vi "RST.vi"(0 "System no.":i32=1 min=1 max=4 step=1, 2 "Axes to be restored":string[](array[string]), 3 "All axes?":bool, 4 "Axis identifier?":bool=TRUE, 5 "error in":errorcluster) -> (19 "error out":errorcluster)   [LabVIEW 2020]
doc: "Restores parameters or resets E-816 master unit.\n\nC-702: If All axes = TRUE, then Axis identifier must be TRUE. Restores last saved stage configuration in volatile memeory (RAM) for any of the specified axes. Loads back the stage configuration (can be modified with CST) and the motion parameters (can be modified with SPA) which were last saved with SAV. \n\nC-848: If All axes = TRUE, then Axis identifier must be TRUE. Restores parameters of any of the specified axes which have been modified using SPA command to values from last SAV.\nC-880: If All axes = TRUE, then Axis identifier must be TRUE. Restores parameters of any of the specified axes which have been modified using SPA command to values from last SAV. \nE-816: All axes = TRUE, Axis identifier = FALSE; this command affects the master unit only. (Resets the master unit.)"
panel:
  # "Restores parameters or resets E-816 master unit."
  # "If all axes: use"
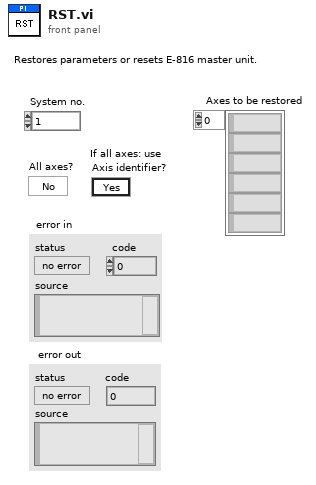
[diagram p1: front panel]
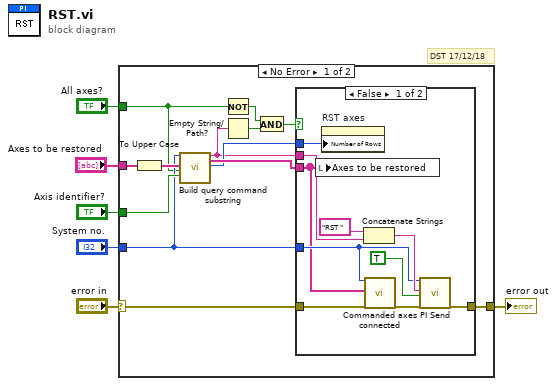
[diagram p0: block diagram]
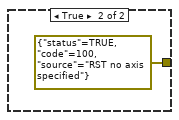
[diagram p2: hidden frame]
diagram:
  # "DST 17/12/18"
  n1 = case shown="No Error" "error in" {
    selector: "error in" -> [w10 w31]
    tunnel: "Axes to be restored" -> [w19 _]
    tunnel: "Axis identifier?" -> [w17 _]
    tunnel: "System no." -> [w16 _]
    tunnel: "All axes?" -> [w13 _]
    tunnel: [w11 w31] -> w2
    frame No Error {
      n2 = To Upper Case(1:w19) -> (0:w18:string[])
      n3 = call "Build query command substring.vi"("System no."=w16, "Axes to query in"=w18, "Query\nAll axes?"=w13, "For all axes: use\nAxis identifier?"=w17) -> ("Command substring"=w7:string, "Axes to query out"=w15:string[], "Number of rows"=w14:u32)  [unwired: 2 in, 11 out]
      n4 = Not(x=w13) -> (.not. x?=w12:bool)
      n5 = Empty String/Path?(string/path=w7) -> (empty?=w8:bool)
      n6 = And(x=w12, y=w8) -> (x .and. y?=w9:bool)
      n7 = case shown="False" w9 {
        tunnel: w7 -> [w26 _]
        tunnel: w16 -> [w25 _]
        tunnel: w15 -> [w24 _]
        tunnel: w14 -> [w22 _]
        tunnel: [w21 errorcluster {"status"=TRUE, "code"=100, "source"="RST no axis specified"} ("error out")] -> w11
        tunnel: w10 -> [w20 _]
        frame False {
          n8 = local write "Axes to be restored"(w24) -> ()
          n9 = property on="RST axes" class="Arr (strict)"("Number of Rows"=w22) -> ()  [unwired: 2 in, 2 out]
          n10 = Concatenate Strings("RST ", w26) -> (w27:string)
          n11 = call "Commanded axes connected.vi"("System no."=w25, "Commanded axes"=w24, "error in"=w20) -> ("error out"=w23:errorcluster)  [unwired: 1 in, 15 out]
          n12 = call "PI Send.vi"("System no."=w25, "String to send"=w27, "Attach termination char.?"=TRUE ("Attach Linefeed?"), "error in"=w23) -> ("error out"=w21:errorcluster)  [unwired: 2 in, 13 out]
        }
        frame True {
        }
      }
    }
    frame Error {
    }
  }
  "error out" <- w2
